vi "Write Perimeter.vi"(8 "error in (no error)":errorcluster, 10 "Perimeter":dbl, 11 "Circle in":refnum<class "Circle.lvclass">) -> (0 "error out":errorcluster, 3 "Circle out":refnum<class "Circle.lvclass">)   [LabVIEW 2015]
uses:
  Circle.lvclass
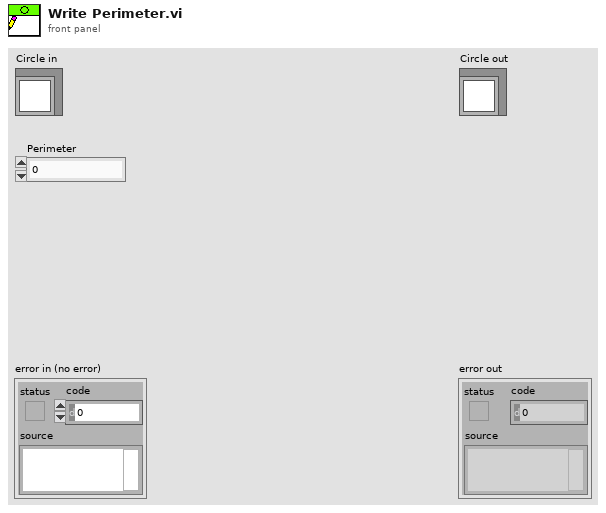
[diagram p1: front panel]
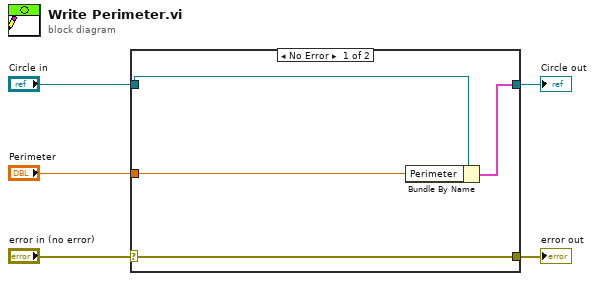
[diagram p0: block diagram]
diagram:
  n1 = case shown="No Error" "error in (no error)" {
    selector: "error in (no error)" -> [w9 w10]
    tunnel: [w9 w10] -> w4
    tunnel: [w7 w11] -> w2
    tunnel: "Circle in" -> [w8 w11]
    tunnel: "Perimeter" -> [w6 _]
    frame No Error {
      n2 = Bundle By Name(cluster=w8, "Perimeter"=w6) -> (w7:cluster{})
    }
    frame Error {
    }
  }
  "error out" <- w4
  "Circle out" <- w2
